vi "Generate Velocity Vectors.vi"(9 "Nonholonomic Headings":cluster{dbl[]}[](array[cluster]), 11 "Trajectory Data In":T1(array[cluster])) -> (3 "Trajectory Data Out":T3(array[cluster]))   [LabVIEW 2025]
uses:
  Types/Segment Type.ctl
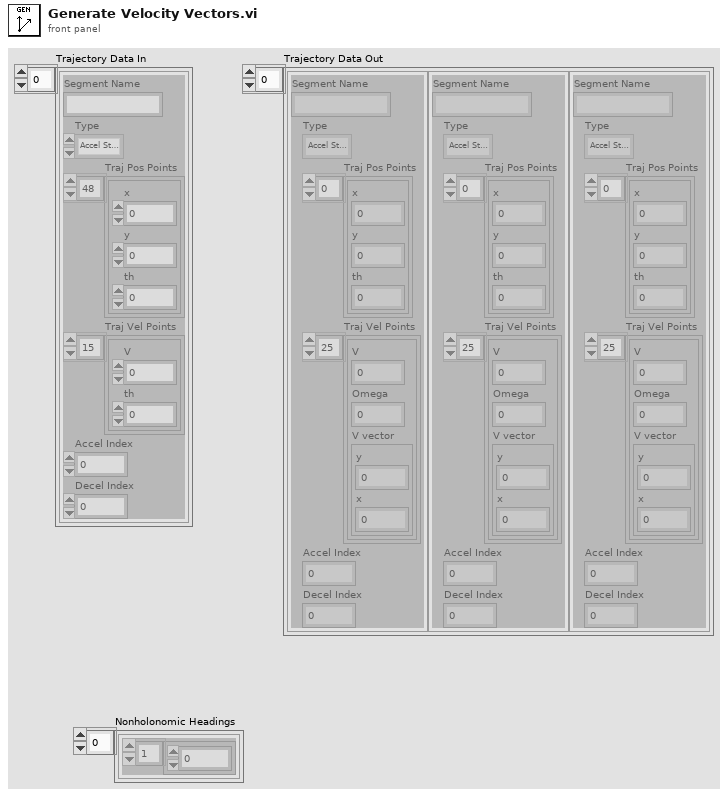
[diagram p1: front panel]
types:
  T1 = cluster{"Segment Name":string, "Type":enum16{"Accel Straight", "Const Straight", "Blend", "Circle"}, "Traj Pos Points":cluster{"x":dbl, "y":dbl, "th":dbl}[], "Traj Vel Points":cluster{"V":dbl, "th":dbl}[], "Accel Index":i32, "Decel Index":i32}[]
  T2 = typedef "Segment Type.ctl" = enum16{"Accel Straight", "Const Straight", "Blend", "Circle", "Bezier"}
  T3 = cluster{"Segment Name":string, "Type":T2, "Traj Pos Points":cluster{"x":dbl, "y":dbl, "th":dbl}[], "Traj Vel Points":cluster{"V":dbl, "Omega":dbl, "V vector":cluster{"y":dbl, "x":dbl}}[], "Accel Index":i32, "Decel Index":i32}[]
  T4 = cluster{"Segment Name":string, "Type":T2, "Traj Pos Points":cluster{"x":dbl, "y":dbl, "th":dbl}[], "Traj Vel Points":cluster{"V":dbl, "Omega":dbl, "V vector":cluster{"y":dbl, "x":dbl}}[], "Accel Index":i32, "Decel Index":i32}
  T5 = enum16{"Accel Straight", "Const Straight", "Blend", "Circle"}
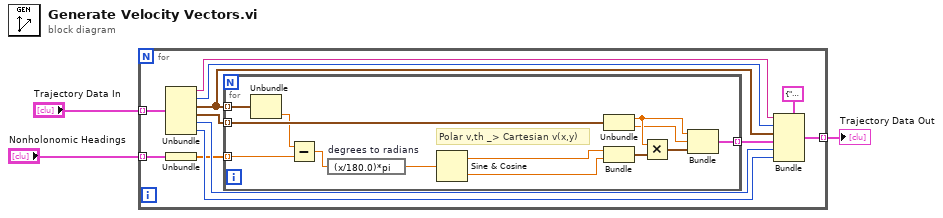
[diagram p0: block diagram]
diagram:
  n1 = for {
    tunnel: "Trajectory Data In" -> [w5] mode=indexing
    tunnel: [w14] -> w3 mode=indexing
    tunnel: "Nonholonomic Headings" -> [w4] mode=indexing
    n2 = Unbundle(w5) -> ("Segment Name"=w13:string, "Type"=w12:T5, "Traj Pos Points"=w6:cluster{"x":dbl, "y":dbl, "th":dbl}[], "Traj Vel Points"=w9:cluster{"V":dbl, "th":dbl}[], "Accel Index"=w11:i32, "Decel Index"=w10:i32)
    n3 = Unbundle(w4) -> (w7:dbl[])
    n4 = for {
      tunnel: w9 -> [w28] mode=indexing
      tunnel: w7 -> [w20] mode=indexing
      tunnel: [w24] -> w8 mode=indexing
      tunnel: w6 -> [w19] mode=indexing
      # "Polar v,th _> Cartesian v(x,y)"
      n5 = Unbundle(w19) -> ("th"=w18:dbl)  [unwired: 2 out]
      n6 = Subtract(x=w18, y=w20) -> (x-y=w21:dbl)
      n7 = expression code="(x/180.0)*pi" "degrees to radians"(w21) -> (w22:dbl)
      n8 = Sine & Cosine(0:w22) -> (1:w16:dbl, 2:w17:dbl)
      n9 = Unbundle(w28) -> ("V"=w26:dbl, "th"=w25:dbl)
      n10 = Bundle(w16, w17) -> (w27:cluster{dbl, dbl})  [unwired: 1 in]
      n11 = Multiply(x=w26, y=w27) -> (x*y=w23:cluster{dbl, dbl})
      n12 = Bundle("V"=w26, "th"=w25, w23) -> (w24:cluster{"V":dbl, "th":dbl, cluster{dbl, dbl}})  [unwired: 1 in]
    }
    n13 = Bundle(cluster=T4 {"Segment Name"="", "Type"=enum."Accel Straight", "Traj Pos Points"=[], "Traj Vel Points"=[], "Accel Index"=0, "Decel Index"=0} ("Trajectory Segment"), "Segment Name"=w13, "Type"=w12, "Traj Pos Points"=w6, "Traj Vel Points"=w8, "Accel Index"=w11, "Decel Index"=w10) -> (w14:T4)
  }
  "Trajectory Data Out" <- w3
